vi "Top Hat SLM.vi"(2 "Action":u16(ring) items=["Read", "Initialize"]) -> (8 "Top hat":dbl[][](array[numeric]))   [LabVIEW 2014]
panel:
  out "Top Hat Radius":dbl
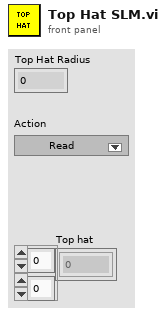
[diagram p1: front panel]
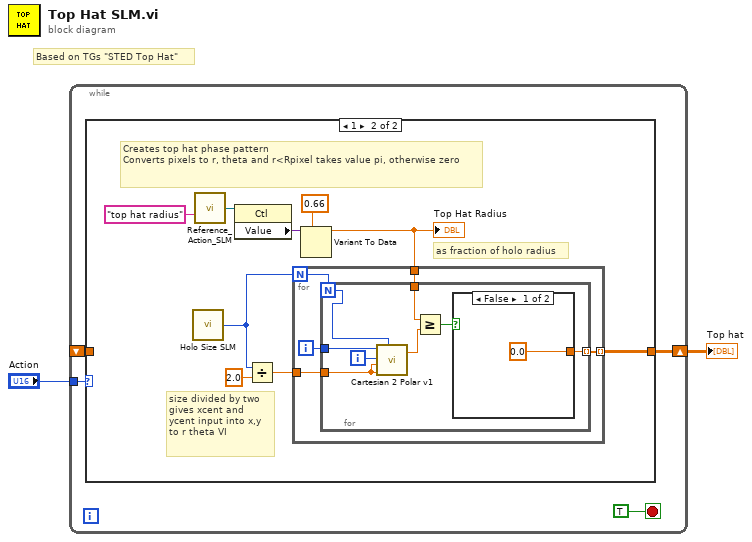
[diagram p0: block diagram]
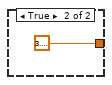
[diagram p3: hidden frame]
diagram:
  # "Based on TGs \"STED Top Hat\""
  n1 = while {
    shift-right: [w4] -> w1
    shift-left: _ -> [w3]
    tunnel: "Action" -> [w5]
    stop <- TRUE stop-if-true
    n2 = case shown="1" w5 {
      tunnel: [w7 w15] -> w4
      tunnel: w3 -> [w7 _]
      frame 0, Default {
      }
      frame 1 {
        # "as fraction of holo radius"
        # "Creates top hat phase pattern\nConverts pixels to r, theta and r<Rpixel takes value pi, otherwise zero"
        # "size divided by two gives xcent and ycent input into x,y to r theta VI"
        n3 = call "Holo Size SLM.vi"() -> ("data"=w13:i32)  [unwired: 15 in]
        n4 = call "Reference_Action_SLM.vi"("Control Name"="top hat radius") -> ("Ref OUT"=w11:refnum<vi>)  [unwired: 12 in, 2 out]
        n5 = property class="Ctl"(reference=w11) -> ("Value"=w10:variant)  [unwired: 1 in, 2 out]
        n6 = Divide(x=w13, y=2.0) -> (x/y=w14:dbl)
        n7 = Variant To Data(type=0.66, Variant=w10) -> (data=w8:dbl)  [unwired: 1 in, 1 out]
        "Top Hat Radius" <- w8
        n8 = for {
          N: w13 -> [w18]
          tunnel: [w20] -> w15 mode=indexing
          tunnel: w14 -> [w19]
          tunnel: w8 -> [w17]
          i -> [w21]
          n9 = for {
            N: w18 -> [w24]
            tunnel: w21 -> [w28]
            tunnel: [w23] -> w20 mode=indexing
            tunnel: w19 -> [w25]
            tunnel: w17 -> [w22]
            i -> [w29]
            n10 = call "Cartesian 2 Polar v1.vi"("x"=w28, "y"=w29, "xcent"=w25, "ycent"=w25, "diam"=w24) -> ("r"=w26:dbl)  [unwired: 1 out]
            n11 = Greater Or Equal?(x=w22, y=w26) -> (x >= y?=w27:bool)
            n12 = case shown="False" w27 {
              tunnel: [0.0 ("zernike") 3.141592653589793] -> w23
              frame False {
              }
              frame True {
              }
            }
          }
        }
      }
    }
  }
  "Top hat" <- w1
